vi "Read Error Data.vi"(8 "error in (no error)":errorcluster, 11 "VISA resource name":refnum<visa-resource-name>) -> (0 "error out":errorcluster, 1 "Error Unit (0: Threshold 1000)":i32(ring) items=["No Result"=-1, "Threshold 1000"=0, "Threshold 100"=1, "Threshold 10"=2, "Parts-per-million"=3, "Percent"=4], 2 "Error":dbl, 3 "VISA resource name out":refnum<visa-resource-name>)   [LabVIEW 2012, in "Fluke 5080.lvlib"]
doc: "Reads the error data between reference value and edit value."
uses:
  <instrlib>/Fluke 5080/Fluke 5080.lvlib
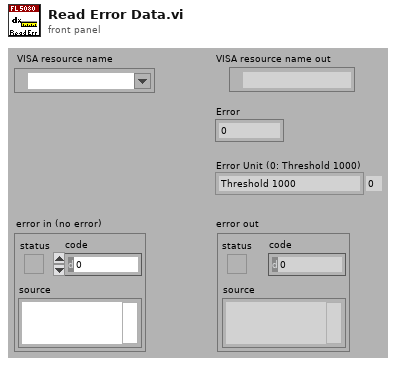
[diagram p1: front panel]
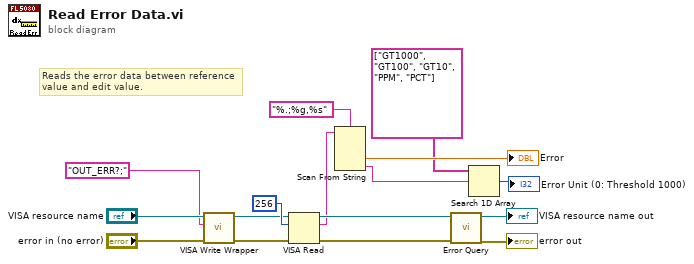
[diagram p0: block diagram]
diagram:
  # "Reads the error data between reference \nvalue and edit value."
  n1 = call <instrlib>:"VISA Write Wrapper.vi"("error in (no error)"="error in (no error)", "Write Buffer"="OUT_ERR?;", "VISA resource name"="VISA resource name") -> ("error out"=w4:errorcluster, "VISA resource name out"=w5:refnum<visa-resource-name>)  [unwired: 7 out]
  n2 = VISA Read(VISA resource name=w5, byte count=u32 256, error in (no error)=w4) -> (VISA resource name out=w14:refnum<visa-resource-name>, read buffer=w11:string, error out=w13:errorcluster)  [unwired: 1 out]
  n3 = Scan From String(format string="%.;%g,%s", input string=w11) -> (output 1=→"Error":dbl, output 2=w7:string)  [unwired: 2 in, 5 out]
  n4 = call <instrlib>:"Error Query.vi"("error in (no error)"=w13, "VISA resource name"=w14) -> ("error out"=→"error out":errorcluster, "VISA resource name out"=→"VISA resource name out":refnum<visa-resource-name>)  [unwired: 8 out]
  n5 = Search 1D Array(1D array=string[] ["GT1000", "GT100", "GT10", "PPM", "PCT"], element=w7) -> (index of element=→"Error Unit (0: Threshold 1000)":i32)  [unwired: 1 out]
